vi "TC to PGSQL.vi"(5 "Calibration":refnum<vi>[](array[refnum]), 6 "I":dbl[](array[numeric]), 7 "AVS names":T2, 8 "error in (no error)":errorcluster, 9 "T":dbl[](array[numeric]), 10 "R":dbl[](array[numeric]), 11 "Inst.TC":refnum<class "Inst.TC.lvclass">) -> (0 "error out":errorcluster, 2 "GetAll":T1, 3 "Inst.TC out":refnum<class "Inst.TC.lvclass">)   [LabVIEW 2019, in "Inst.TC.lvclass"]
uses:
  Inst.TC.lvclass
  Typedefs/Inst.TC.getAll--Cluster.ctl
  C:/Program Files (x86)/National Instruments/LabVIEW 2019/user.lib/LevyLab/Instrument Framework/Instrument/Instrument.lvclass
  Inst.TC.lvclass/Inst.TC.ctl
  FP-TC-Shared/FP-TC-Shared.lvclass
  <userlib>/LevyLab/Instrument Framework/Instrument/Instrument.lvclass
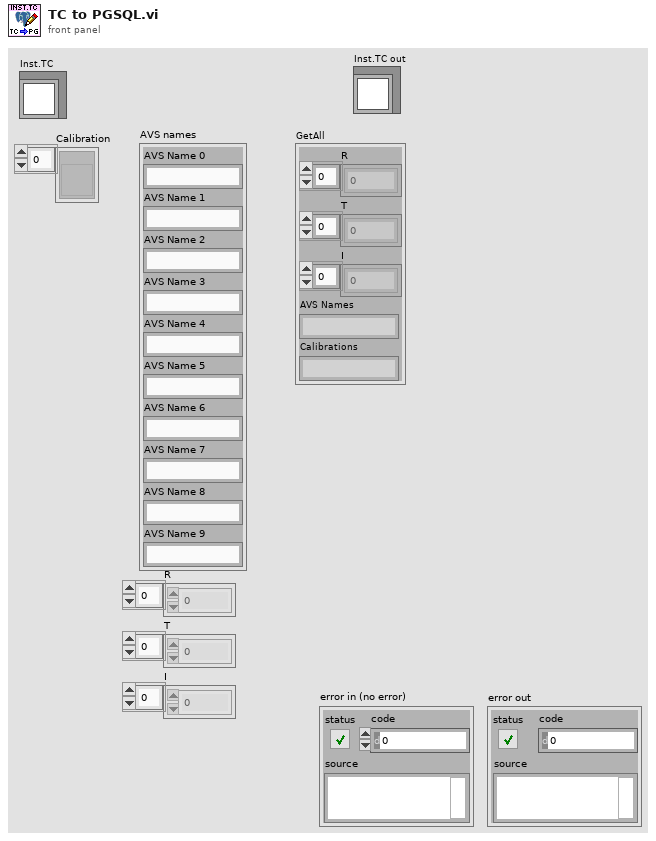
[diagram p1: front panel]
types:
  T1 = typedef "Inst.TC.lvclass/Inst.TC.getAll--Cluster.ctl" = cluster{"R":dbl[], "T":dbl[], "I":dbl[], "AVS Names":string, "Calibrations":string}
  T2 = cluster{"AVS Name 0":string, "AVS Name 1":string, "AVS Name 2":string, "AVS Name 3":string, "AVS Name 4":string, "AVS Name 5":string, "AVS Name 6":string, "AVS Name 7":string, "AVS Name 8":string, "AVS Name 9":string}
  T3 = typedef "FP-TC-Shared.lvclass/LC Type--Enum.ctl" = enum16{"CF_FP", "CF_TC", "CF_TC_Z", "MNK_FP", "MNK_TC", "MNK_TC_Z", "unknown"}
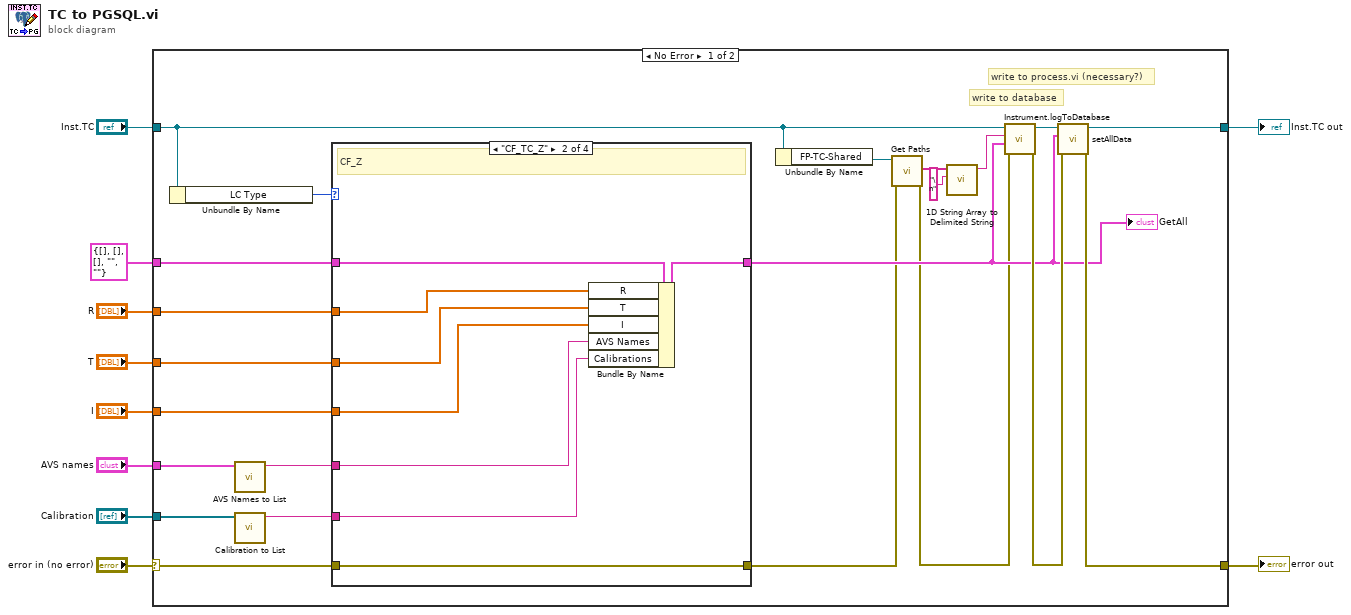
[diagram p0: block diagram]
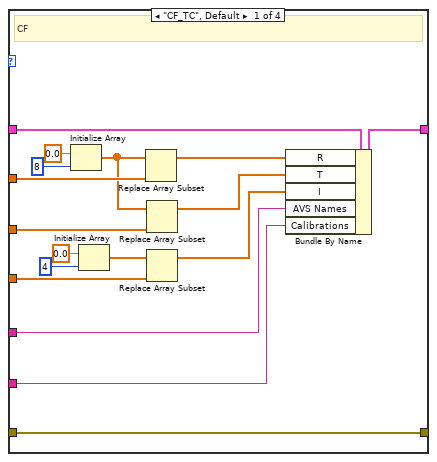
[diagram p2: hidden frame]
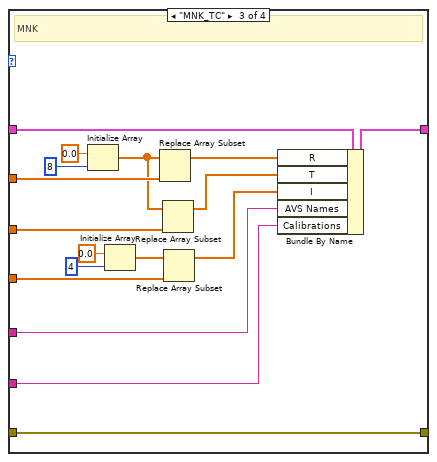
[diagram p3: hidden frame]
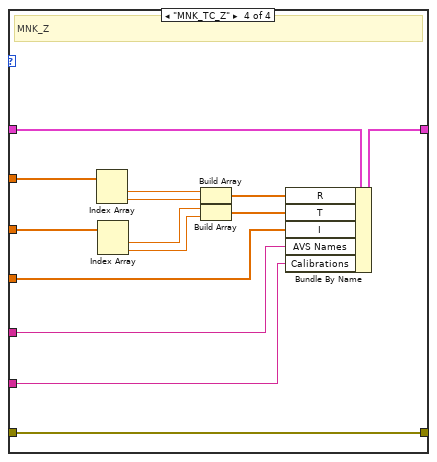
[diagram p4: hidden frame]
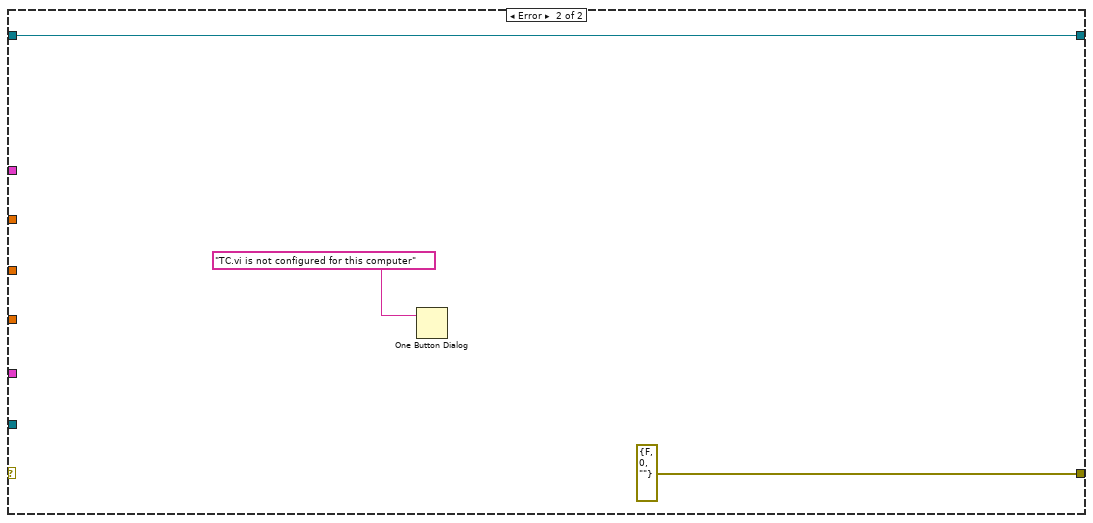
[diagram p5: hidden frame]
diagram:
  n1 = case shown="No Error" "error in (no error)" {
    selector: "error in (no error)" -> [w29 _]
    tunnel: "R" -> [w32 _]
    tunnel: "T" -> [w31 _]
    tunnel: "I" -> [w30 _]
    tunnel: [w20 errorcluster {"status"=FALSE, "code"=0, "source"=""} ("error IO")] -> w1
    tunnel: T1 {"R"=[], "T"=[], "I"=[], "AVS Names"="", "Calibrations"=""} ("GetAll") -> [w28 _]
    tunnel: "Calibration" -> [w27 _]
    tunnel: "AVS names" -> [w26 _]
    tunnel: "Inst.TC" -> [w15 w89]
    tunnel: [w19 w89] -> w2
    frame No Error {
      # "write to database"
      # "write to process.vi (necessary?)"
      n2 = Unbundle By Name(w15) -> ("LC Type"=w23:T3)
      n3 = call "AVS Names to List.vi"("AVS names"=w26) -> ("List"=w24:string)  [unwired: 9 in, 1 out]
      n4 = call "Calibration to List.vi"("Calibration"=w27) -> ("List"=w25:string)  [unwired: 9 in, 1 out]
      n5 = case shown="\"CF_TC_Z\"" w23 {
        tunnel: w32 -> [w42 w56 w69 w85]
        tunnel: w31 -> [w40 w55 w68 w84]
        tunnel: w30 -> [w43 w54 w67 w81]
        tunnel: w24 -> [w36 w53 w61 w83]
        tunnel: w25 -> [w35 w52 w60 w82]
        tunnel: w29 -> [w49 w57 w74 w86]
        tunnel: [w49 w57 w74 w86] -> w14
        tunnel: [w33 w50 w58 w75] -> w18
        tunnel: w28 -> [w34 w51 w59 w76]
        frame "CF_TC", Default {
          # "CF"
          n6 = Initialize Array(0.0 ("element"), 8 ("dimension size")) -> (w41:dbl[])
          n7 = Initialize Array(0.0 ("element"), 4 ("dimension size")) -> (w44:dbl[])
          n8 = Replace Array Subset(array=w41, new element=w42) -> (w39:dbl[])  [unwired: 1 in]
          n9 = Replace Array Subset(array=w41, new element=w40) -> (w38:dbl[])  [unwired: 1 in]
          n10 = Replace Array Subset(array=w44, new element=w43) -> (w37:dbl[])  [unwired: 1 in]
          n11 = Bundle By Name(cluster=w34, "R"=w39, "T"=w38, "I"=w37, "AVS Names"=w36, "Calibrations"=w35) -> (w33:T1)
        }
        frame "CF_TC_Z" {
          # "CF_Z"
          n12 = Bundle By Name(cluster=w51, "R"=w56, "T"=w55, "I"=w54, "AVS Names"=w53, "Calibrations"=w52) -> (w50:T1)
        }
        frame "MNK_TC" {
          # "MNK"
          n13 = Initialize Array(0.0 ("element"), 8 ("dimension size")) -> (w65:dbl[])
          n14 = Initialize Array(0.0 ("element"), 4 ("dimension size")) -> (w70:dbl[])
          n15 = Replace Array Subset(array=w65, new element=w69) -> (w64:dbl[])  [unwired: 1 in]
          n16 = Replace Array Subset(array=w65, new element=w68) -> (w63:dbl[])  [unwired: 1 in]
          n17 = Replace Array Subset(array=w70, new element=w67) -> (w62:dbl[])  [unwired: 1 in]
          n18 = Bundle By Name(cluster=w59, "R"=w64, "T"=w63, "I"=w62, "AVS Names"=w61, "Calibrations"=w60) -> (w58:T1)
        }
        frame "MNK_TC_Z" {
          # "MNK_Z"
          n19 = Index Array(array=w85) -> (element #1=w88:dbl, element #2=w87:dbl)  [unwired: 2 in]
          n20 = Index Array(array=w84) -> (element #1=w79:dbl, element #2=w78:dbl)  [unwired: 2 in]
          n21 = Build Array(w88, w87) -> (w80:dbl[])
          n22 = Build Array(w79, w78) -> (w77:dbl[])
          n23 = Bundle By Name(cluster=w76, "R"=w80, "T"=w77, "I"=w81, "AVS Names"=w83, "Calibrations"=w82) -> (w75:T1)
        }
      }
      "GetAll" <- w18
      n24 = Unbundle By Name(w15) -> ("FP-TC-Shared"=w17:refnum<class "FP-TC-Shared.lvclass">)
      n25 = call-dynamic "Get Paths.vi"("error in (no error)"=w14, "FP-TC-Shared in"=w17) -> ("error out"=w12:errorcluster, "Paths"=w16:string[])  [unwired: 7 in, 1 out]
      n26 = call <vilib>:"1D String Array to Delimited String.vi"("delimiter"="\n", "string array"=w16) -> ("delimited string"=w11:string)  [unwired: 9 in]
      n27 = call <userlib>:"Instrument.logToDatabase.vi"("error in (no error)"=w12, "Data"=w18, "Paths"=w11, "Instrument"=w15) -> ("error out"=w21:errorcluster, "Instrument out"=w22:refnum<class "Inst.TC.lvclass">)  [unwired: 6 in]
      n28 = call <userlib>:"setAllData.vi"("error in (no error)"=w21, "AllData"=w18, "Instrument in"=w22) -> ("error out"=w20:errorcluster, "Instrument out"=w19:refnum<class "Inst.TC.lvclass">)  [unwired: 7 in]
    }
    frame Error {
      n29 = One Button Dialog(message="TC.vi is not configured for this computer" ("URL")) -> ()  [unwired: 1 in, 1 out]
    }
  }
  "error out" <- w1
  "Inst.TC out" <- w2
